vi "HalfAdder.vi"(10 "b":bool, 11 "a":bool) -> (2 "carry":bool, 3 "sum":bool)   [LabVIEW 2014]
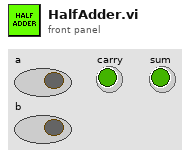
[diagram p1: front panel]
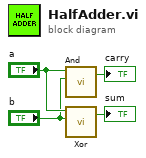
[diagram p0: block diagram]
diagram:
  n1 = call "And.vi"("b"="b", "a"="a") -> ("out"=→"carry":bool)  [unwired: 3 in]
  n2 = call "Xor.vi"("b"="b", "a"="a") -> ("out"=→"sum":bool)  [unwired: 3 in]
